vi "cleaner.vi"() -> ()   [LabVIEW 2019]
uses:
  fbda3c1a-45bc-4ffe-ae8e-6074ddd48b06.vi
panel:
  out "map":map{u32, u32}(c390)
  out "sorted 2D array":i32[][](array[numeric])
  out "Array":i32[][](array[numeric])
  out "Counts (map)":map{u32, u32}(c390)
  in  "Read Array":string[](array[string])
  in  "Delimiter (\\n)":string="\n"
  in  "Raw Response":string
  out "appended array":u32[][](array[numeric])
  out "Channel":u32[](array[numeric])
  out "Energy":u32[](array[numeric])
  out "Chan+Energy":u32[](array[numeric])
  out "Clk Ticks":u32[](array[numeric])
  out "Sr No":u32[](array[numeric])
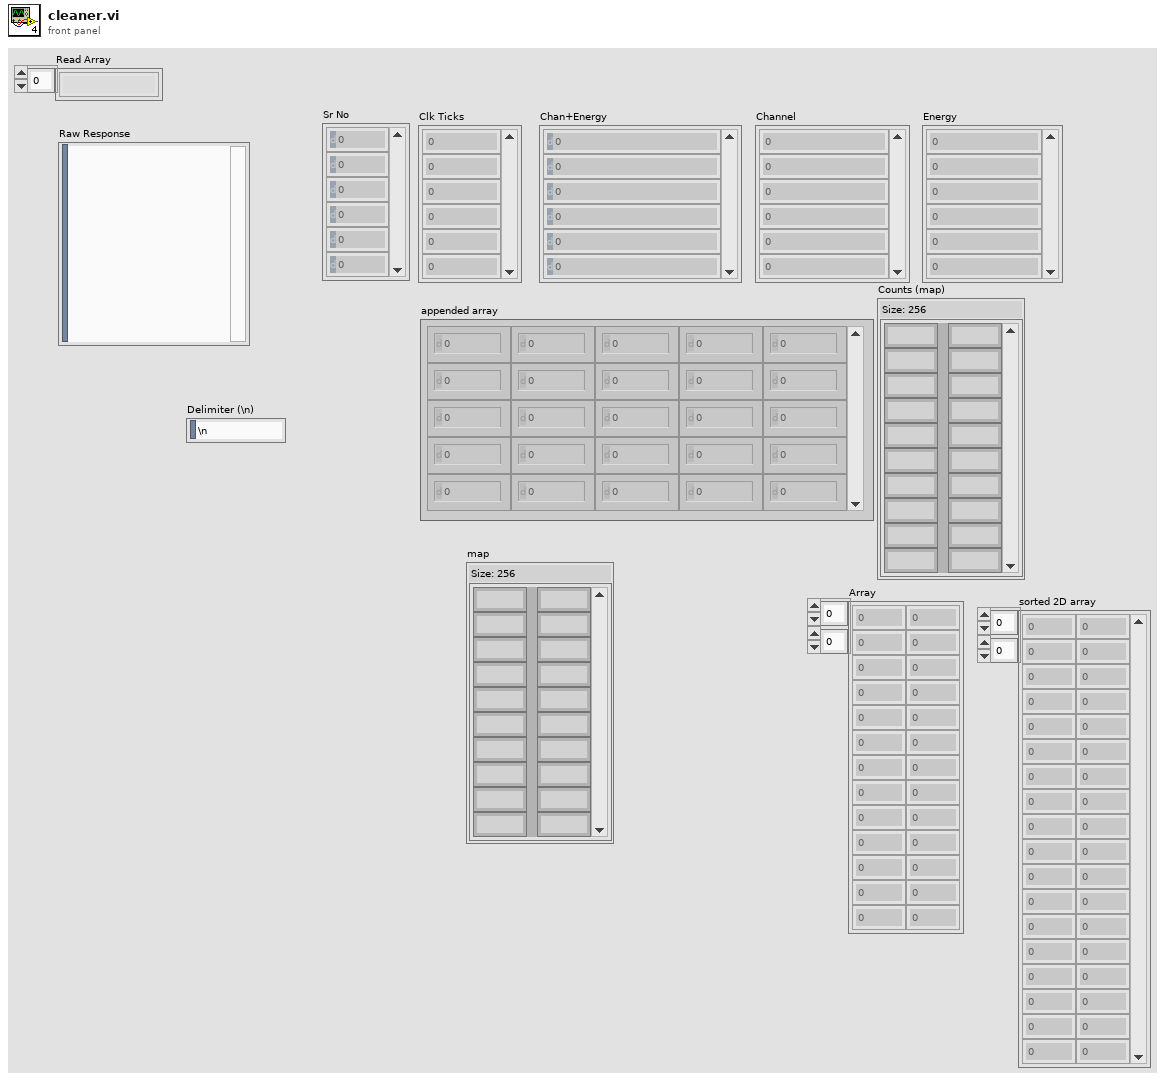
[diagram p1: front panel]
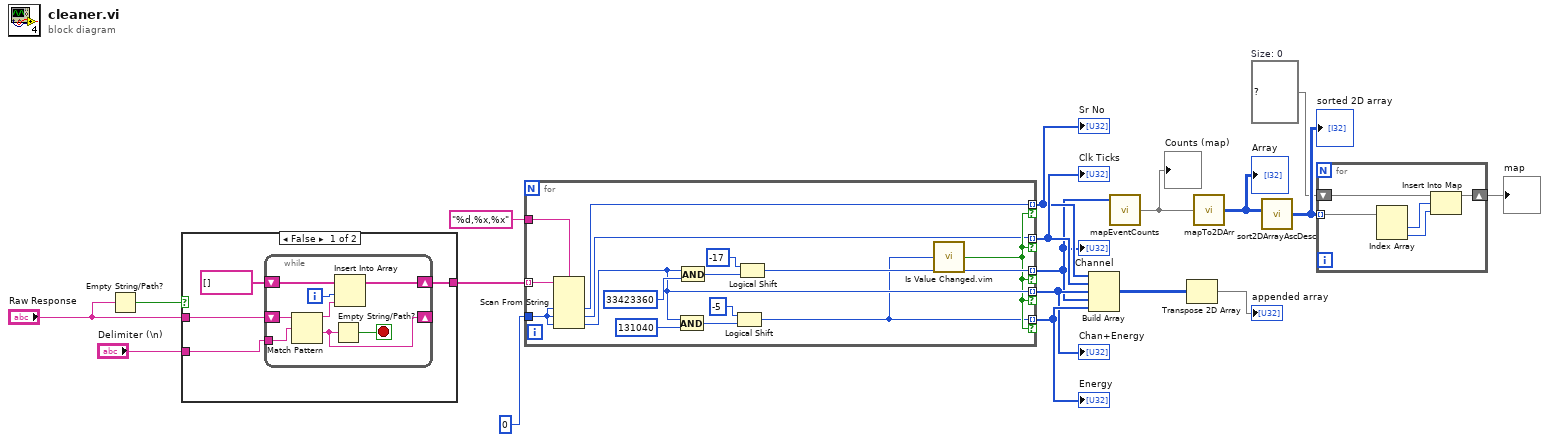
[diagram p0: block diagram]
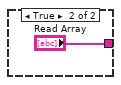
[diagram p2: hidden frame]
diagram:
  w2 = map{u32, u32} {}  # Size: 0
  n1 = Empty String/Path?(string/path="Raw Response") -> (empty?=w7:bool)
  n2 = case shown="False" w7 {
    tunnel: "Delimiter (\\n)" -> [w21 _]
    tunnel: [w20 "Read Array"] -> w9
    tunnel: "Raw Response" -> [w19 _]
    frame False {
      n3 = while {
        tunnel: w21 -> [w29]
        shift-right: [w26] -> _
        shift-left: w19 -> [w30]
        shift-right: [w27] -> w20
        shift-left: string[] [] -> [w28]
        i -> [w23]
        stop <- w25 stop-if-true
        n4 = Match Pattern(string=w30, regular expression=w29) -> (before substring=w24:string, after substring=w26:string)  [unwired: 1 in, 2 out]
        n5 = Empty String/Path?(string/path=w26) -> (empty?=w25:bool)
        n6 = Insert Into Array(array=w28, index=w23, new element=w24) -> (w27:string[])
      }
    }
    frame True {
    }
  }
  n7 = for {
    tunnel: w9 -> [w46] mode=indexing
    tunnel: [w45] -> w11 mode=indexing if=w34
    tunnel: [w33] -> w12 mode=indexing if=w34
    tunnel: [w36] -> w13 mode=indexing if=w34
    tunnel: [w42] -> w6 mode=indexing if=w34
    tunnel: [w32] -> w14 mode=indexing if=w34
    tunnel: "%d,%x,%x" ("format string (%d,%x,%x)") -> [w41]
    tunnel: u32 0 -> [w40]
    n8 = Scan From String(format string=w41, input string=w46, default 1=w40, default 2=w40, default 3=w40) -> (output 1=w45:u32, output 2=w33:u32, output 3=w36:u32)  [unwired: 2 in, 3 out]
    n9 = And(x=w36, y=u32 131040 ("value")) -> (x .and. y?=w35:u32)
    n10 = And(x=w36, y=u32 33423360 ("value")) -> (x .and. y?=w38:u32)
    n11 = Logical Shift(y=-5, x=w35) -> (x << y=w32:u32)
    n12 = Logical Shift(y=-17, x=w38) -> (x << y=w42:u32)
    n13 = call "Is Value Changed.vim"("value"=w32) -> ("changed or first call?"=w34:bool)
  }
  "Sr No" <- w11
  "Clk Ticks" <- w12
  "Chan+Energy" <- w13
  "Energy" <- w14
  "Channel" <- w6
  n14 = Build Array(w11, w12, w13, w6, w14) -> (w15:u32[][])
  n15 = call "mapEventCounts.vi"("Count"=w6) -> ("Counts (map)"=w5:map{u32, u32})  [unwired: 3 in, 1 out]
  "Counts (map)" <- w5
  n16 = Transpose 2D Array(2D array=w15) -> (transposed array=→"appended array":u32[][])
  n17 = call "mapTo2DArr.vi"("Map"=w5) -> ("2D Array"=w4:i32[][])
  "Array" <- w4
  n18 = call "sort2DArrayAscDesc.vi"("2D Array"=w4) -> ("sorted 2D array"=w3:i32[][])  [unwired: 5 in]
  "sorted 2D array" <- w3
  n19 = for {
    tunnel: w3 -> [w49] mode=indexing
    shift-right: [w50] -> w1
    shift-left: w2 -> [w51]
    n20 = Index Array(array=w49) -> (element #1=w48:i32, element #2=w47:i32)  [unwired: 2 in]
    n21 = Insert Into Map(map in=w51, key=w48, value=w47) -> (map out=w50:map{u32, u32})  [unwired: 2 out]
  }
  "map" <- w1
